vi "SetBiasNumber.vi"(1 "Volt":i32 min=0 max=4095, 2 "Type":enum16{"Video", "Clock"}(ring)=enum."Clock", 3 "DAC":i32 min=0 max=15, 4 "Board":i32=2 min=0 max=15) -> (0 "Error":bool)   [LabVIEW 2014]
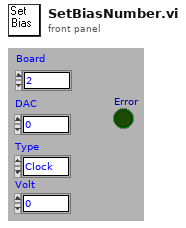
[diagram p1: front panel]
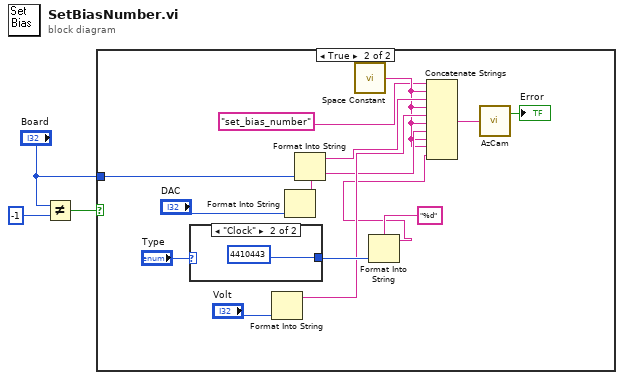
[diagram p0: block diagram]
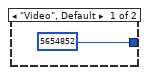
[diagram p3: hidden frame]
diagram:
  n1 = Not Equal?(x="Board", y=-1) -> (x != y?=w2:bool)
  n2 = case shown="True" w2 {
    tunnel: "Board" -> [_ w14]
    frame False {
    }
    frame True {
      n3 = case shown="\"Clock\"" "Type" {
        tunnel: [5654852 4410443] -> w13
        frame "Video", Default {
        }
        frame "Clock" {
        }
      }
      n4 = Format Into String("Volt") -> (resulting string=w10:string)  [unwired: 3 in, 1 out]
      n5 = Format Into String("DAC") -> (resulting string=w9:string)  [unwired: 3 in, 1 out]
      n6 = Format Into String(w14) -> (resulting string=w11:string)  [unwired: 3 in, 1 out]
      n7 = call <vilib>:"Space Constant.vi"() -> ("String"=w8:string)
      n8 = Format Into String(format string="%d" ("Format String"), w13) -> (resulting string=w7:string)  [unwired: 2 in, 1 out]
      n9 = Concatenate Strings("set_bias_number" ("string"), w8, w11, w8, w10, w8, w9, w8, w8, w7) -> (w6:string)
      n10 = call "AzCam.vi"("Command"=w6) -> ("Error"=→"Error":bool)  [unwired: 1 out]
    }
  }
